vi "Initialize mailbox.vi"(8 "error in":errorcluster, 9 "name (unnamed)":string, 11 "MailboxSize(-1)":i32=-1) -> (0 "error out":errorcluster, 3 "Queue out":refnum<queue>)   [LabVIEW 2017]
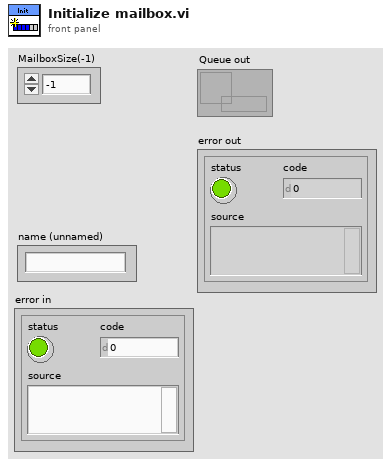
[diagram p1: front panel]
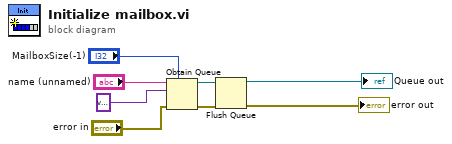
[diagram p0: block diagram]
diagram:
  n1 = Obtain Queue(max queue size (-1, unlimited)="MailboxSize(-1)", name (unnamed)="name (unnamed)", element data type=variant ("Variant"), error in (no error)="error in") -> (queue out=w4:refnum<queue>, error out=w3:errorcluster)  [unwired: 1 in, 1 out]
  n2 = Flush Queue(queue=w4, error in (no error)=w3) -> (queue out=→"Queue out":refnum<queue>, error out=→"error out":errorcluster)  [unwired: 1 out]
